vi "milliGAT Configure and Run Continuous.vi"() -> ()   [LabVIEW 2015]
uses:
  Global FIA milliGAT.lvlib
  Public/Utility/Pump Direction.ctl
  Public/Utility/Pump Address.ctl
panel:
  in  "Flow Parameters":T1={"Peak Flow (uL/s)"=100.0, "Starting Flow (uL/s)"=0.1, "Acceleration (uL/s^2)"=500.0, "Deceleration (uL/s^2)"=500.0}
  in  "Pump ID (0:A)":T2
  in  "Stop":bool
  out "Microliters":dbl
  in  "Direction":T3
  in  "Serial Configuration":cluster{"Baud Rate":u32}={"Baud Rate"=9600} {"Baud Rate" items=["300"=300, "600"=600, "1200"=1200, "2400"=2400, "4800"=4800, "9600"=9600, "19200"=19200]}
  out "error out":errorcluster
  in  "VISA resource name":refnum<visa-resource-name>="COM1"
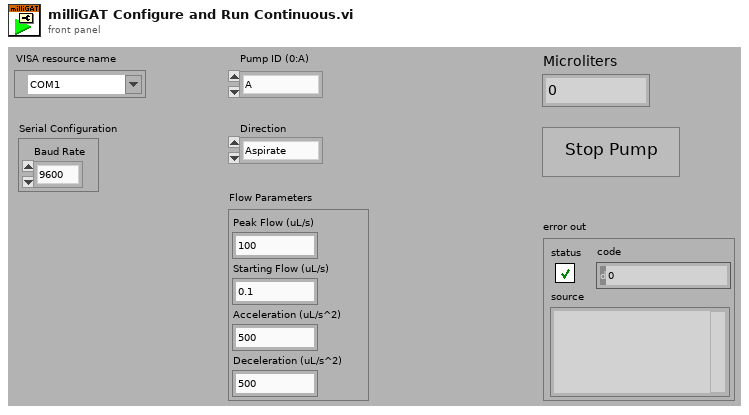
[diagram p1: front panel]
types:
  T1 = cluster{"Peak Flow (uL/s)":dbl, "Starting Flow (uL/s)":dbl, "Acceleration (uL/s^2)":dbl, "Deceleration (uL/s^2)":dbl}
  T2 = typedef "Global FIA milliGAT.lvlib/Pump Address.ctl" = enum16{"A", "B", "C", "D", "E", "F", "G", "H", "I", "J", "K", "L", "M", "N", "O", "P", "Q", "R", "S", "T", "U", "V", "W", "X", "Y", "Z", "a", "b", "c", "d", "e", "f", "g", "h", "i", "j", "k", "l", "m", "n", "o", "p", "q", "r", "s", "t", "u", "v", "w", "x", "y", "z", "0", "1", "2", "3", "4", "5", "6", "7", "8", "9"}
  T3 = typedef "Global FIA milliGAT.lvlib/Pump Direction.ctl" = enum16{"Aspirate", "Dispense"}
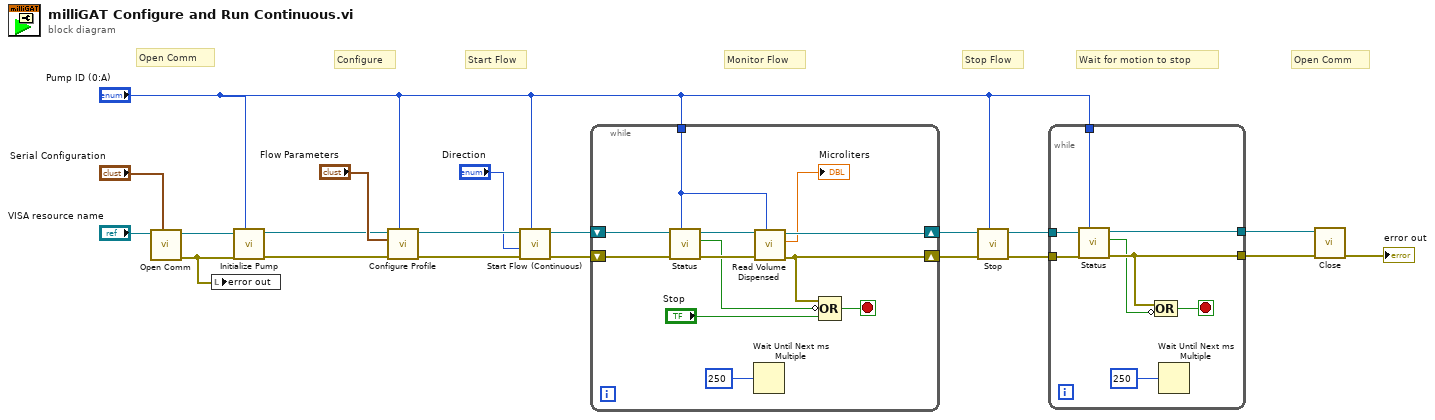
[diagram p0: block diagram]
diagram:
  # "Open Comm"
  # "Stop Flow"
  # "Open Comm"
  # "Start Flow"
  # "Configure"
  # "Monitor Flow"
  # "Wait for motion to stop"
  n1 = call "Open Comm.vi"("Serial Configuration"="Serial Configuration", "VISA resource in"="VISA resource name") -> ("error out"=w4:errorcluster, "VISA resource out"=w12:refnum<visa-resource-name>)  [unwired: 8 in]
  n2 = local write "error out"(w4) -> ()
  n3 = call "Initialize Pump.vi"("Pump ID (0:A)"="Pump ID (0:A)", "error in (no error)"=w4, "VISA resource in"=w12) -> ("error out"=w1:errorcluster, "VISA resource out"=w2:refnum<visa-resource-name>)  [unwired: 7 in]
  n4 = call "Configure Profile.vi"("Pump ID (0:A)"="Pump ID (0:A)", "error in (no error)"=w1, "Flow Parameters"="Flow Parameters", "VISA resource in"=w2) -> ("error out"=w19:errorcluster, "VISA resource out"=w20:refnum<visa-resource-name>)  [unwired: 6 in]
  n5 = call "Start Flow (Continuous).vi"("Pump ID (0:A)"="Pump ID (0:A)", "error in (no error)"=w19, "Direction (0:Aspirate)"="Direction", "VISA resource in"=w20) -> ("error out"=w16:errorcluster, "VISA resource out"=w17:refnum<visa-resource-name>)  [unwired: 6 in]
  n6 = while {
    shift-right: [w32] -> w9
    shift-left: w17 -> [w30]
    tunnel: "Pump ID (0:A)" -> [w29]
    shift-right: [w22] -> w10
    shift-left: w16 -> [w31]
    stop <- w24 stop-if-true
    n7 = call "Status.vi"("Pump ID (0:A)"=w29, "error in (no error)"=w31, "VISA resource in"=w30) -> ("error out"=w26:errorcluster, "moving"=w21:bool, "VISA resource out"=w27:refnum<visa-resource-name>)  [unwired: 6 in]
    n8 = Wait Until Next ms Multiple(millisecond multiple=u32 250) -> ()  [unwired: 1 out]
    n9 = call "Read Volume Dispensed.vi"("Pump ID (0:A)"=w29, "error in (no error)"=w26, "VISA resource in"=w27) -> ("error out"=w22:errorcluster, "microliters"=→"Microliters":dbl, "VISA resource out"=w32:refnum<visa-resource-name>)  [unwired: 6 in]
    n10 = Compound Arithmetic op=OR(w22, invert w21, "Stop") -> (w24:bool)
  }
  n11 = call "Stop.vi"("Pump ID (0:A)"="Pump ID (0:A)", "error in (no error)"=w10, "VISA resource in"=w9) -> ("error out"=w8:errorcluster, "VISA resource out"=w7:refnum<visa-resource-name>)  [unwired: 7 in]
  n12 = while {
    tunnel: w8 -> [w39]
    tunnel: w7 -> [w40]
    tunnel: "Pump ID (0:A)" -> [w38]
    tunnel: [w36] -> w5
    tunnel: [w37] -> w6
    stop <- w34 stop-if-true
    n13 = call "Status.vi"("Pump ID (0:A)"=w38, "error in (no error)"=w39, "VISA resource in"=w40) -> ("error out"=w36:errorcluster, "moving"=w35:bool, "VISA resource out"=w37:refnum<visa-resource-name>)  [unwired: 6 in]
    n14 = Compound Arithmetic op=OR(w36, invert w35) -> (w34:bool)
    n15 = Wait Until Next ms Multiple(millisecond multiple=u32 250) -> ()  [unwired: 1 out]
  }
  n16 = call "Close.vi"("error in (no error)"=w5, "VISA resource in"=w6) -> ("error out"=→"error out":errorcluster)  [unwired: 9 in]
